vi "subXMLFindNode.vi"(7 "Node name":string, 8 "error in (no error)":errorcluster, 9 "Property value":string, 10 "Property name":string, 11 "Refnum in":refnum<k20>) -> (1 "Nodes":refnum<k20>[](array[refnum]), 3 "Refnum":refnum<k20>)   [LabVIEW 2019, in "SolutionBuilder.lvlib" / "SolutionBuilder.lvclass"]
uses:
  SolutionBuilder.lvclass
  <vilib>/xml/NI_XML.lvlib
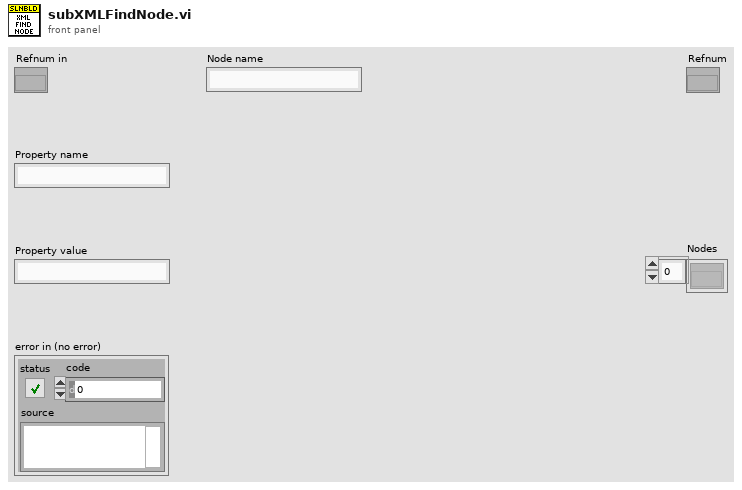
[diagram p1: front panel]
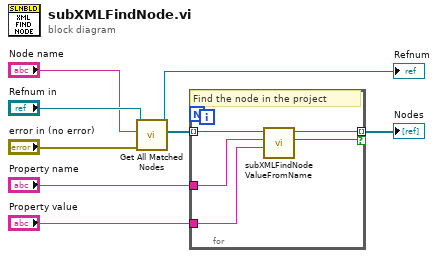
[diagram p0: block diagram]
diagram:
  n1 = call <vilib>:"Get All Matched Nodes.vi"("error in (no error)"="error in (no error)", "XPath expression"="Node name", "node in"="Refnum in") -> ("node result array"=w7:refnum<k20>[], "node out"=→"Refnum":refnum<k20>)  [unwired: 6 in, 1 out]
  n2 = for {
    tunnel: w7 -> [w13] mode=indexing
    tunnel: [w12] -> w1 mode=indexing if=w9
    tunnel: "Property name" -> [w11]
    tunnel: "Property value" -> [w10]
    # "Find the node in the project"
    n3 = call "subXMLFindNodeValueFromName.vi"("Property value"=w10, "Property name"=w11, "Refnum in"=w13) -> ("Found?"=w9:bool, "Refnum out"=w12:refnum<k20>)  [unwired: 6 in, 1 out]
  }
  "Nodes" <- w1
